vi "PIL_GUI_Fake.vi"() -> ()   [LabVIEW 2015]
doc: "Utilisez ce modèle pour construire un modèle de conception Machine à états standard. Chaque état exécute du code et détermine l'état suivant à exécuter."
uses:
  QMH_MessageCluster.ctl
panel:
  in  "Commande onglets":enum32{"Experiment", "Hardware"}(tab)
  out "error out":errorcluster
  in  "error in (no error)":errorcluster
  out "Consumer State":string
  in  "Exit":bool caption="Stop"
  in  "Save":bool caption="Stop"
  in  "Load":bool caption="Stop"
  in  "Stop":bool
  in  "Settings":bool caption="Record"
  in  "Play":bool
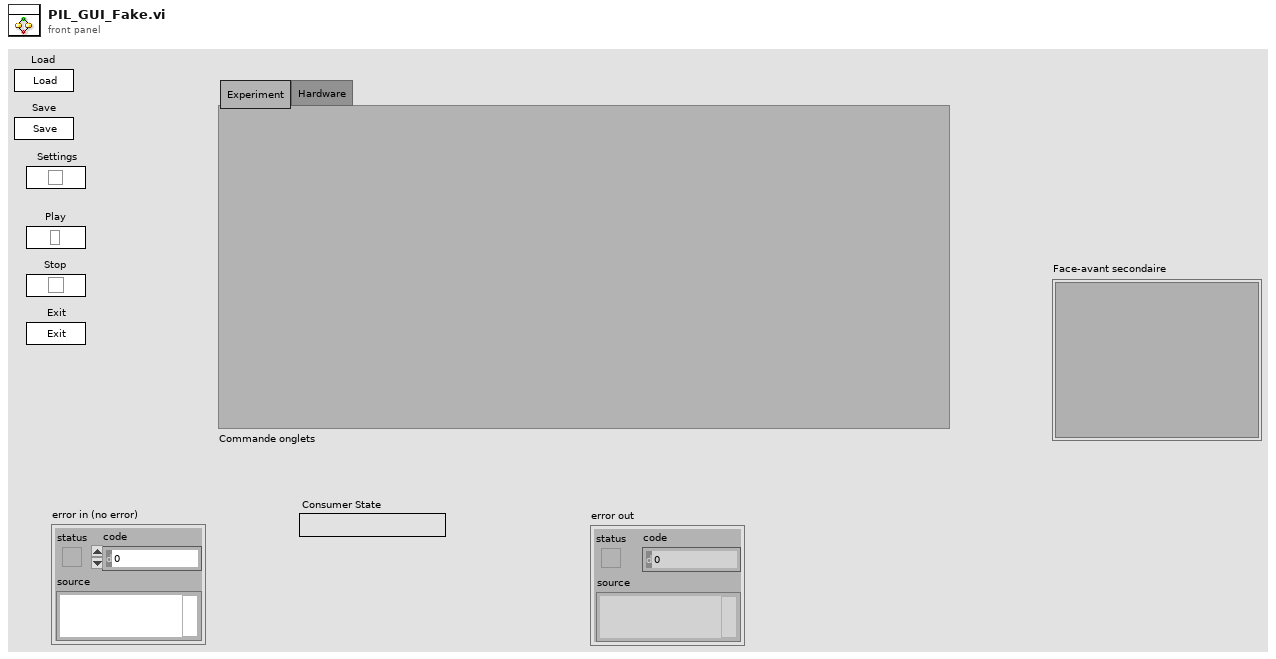
[diagram p1: front panel]
types:
  T1 = enum16{"Initialize", "Settings", "Load", "Save", "Play", "Stop", "Exit"}
  T2 = typedef "QMH_MessageCluster.ctl" = cluster{"Command":enum16{"Initialize", "Settings", "Load", "Save", "Play", "Stop", "Exit"}, "Data":variant}
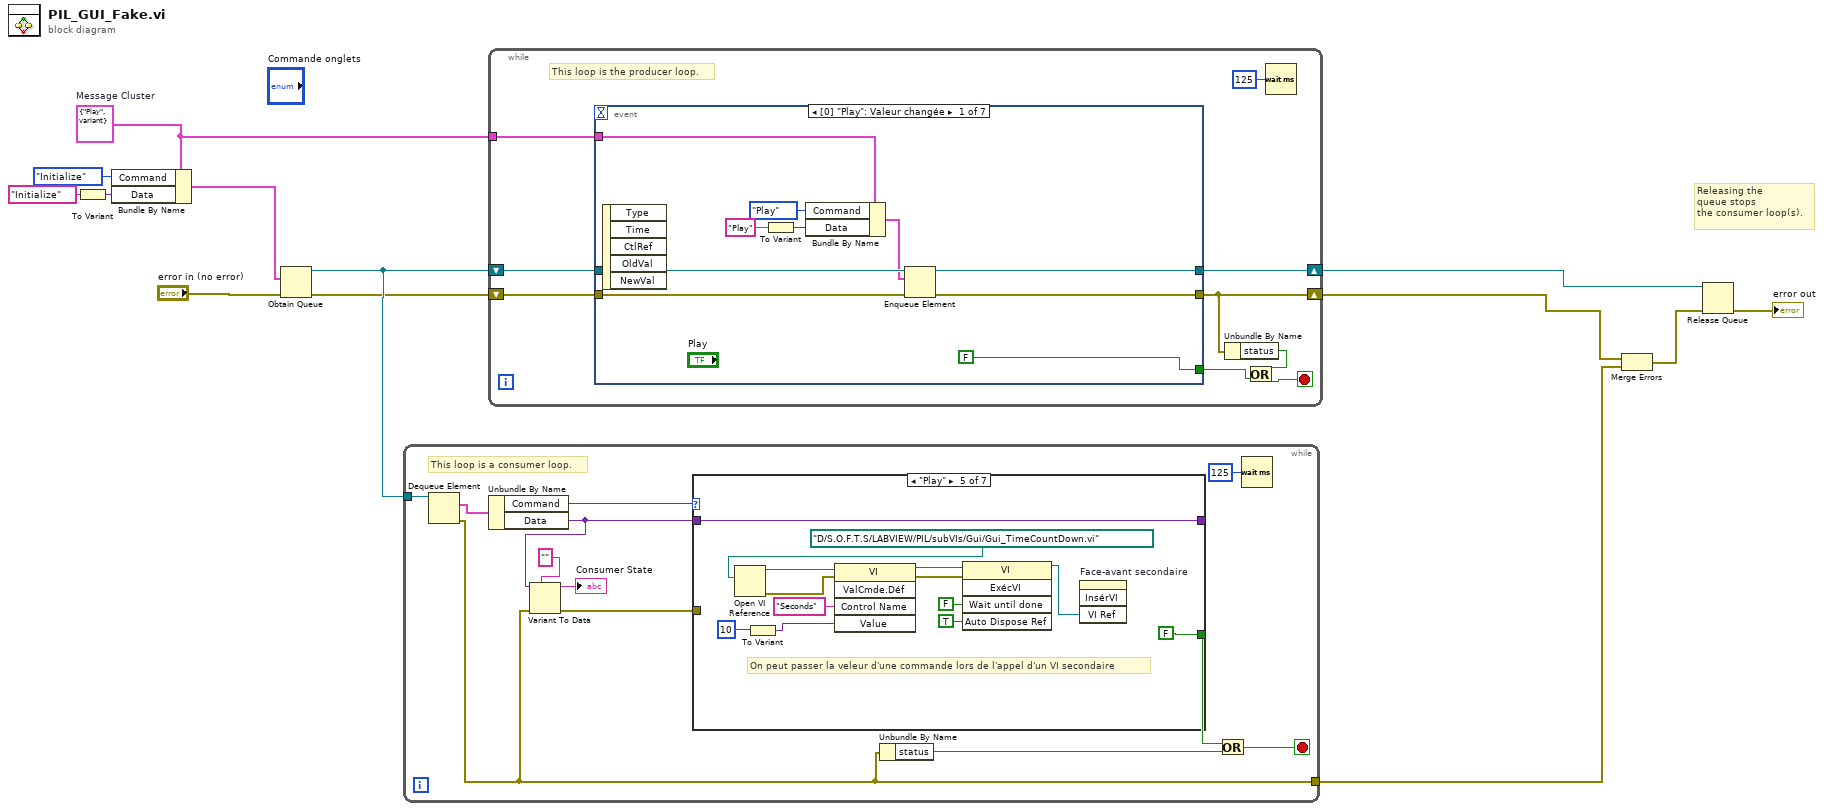
[diagram p0: block diagram]
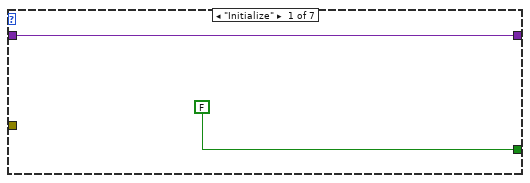
[diagram p2: hidden frame]
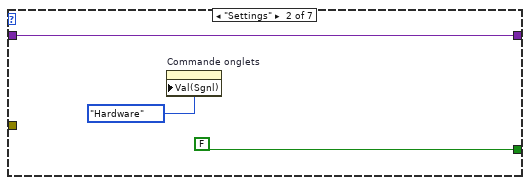
[diagram p3: hidden frame]
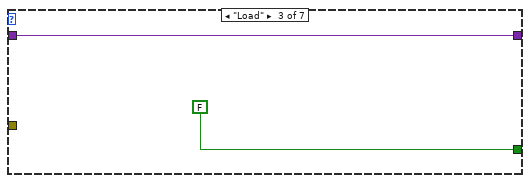
[diagram p4: hidden frame]
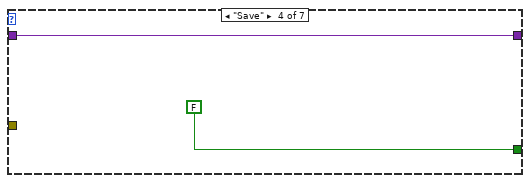
[diagram p5: hidden frame]
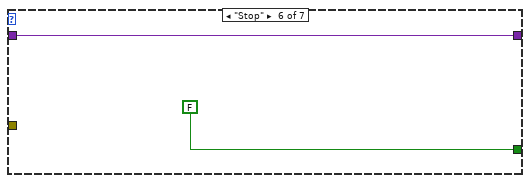
[diagram p6: hidden frame]
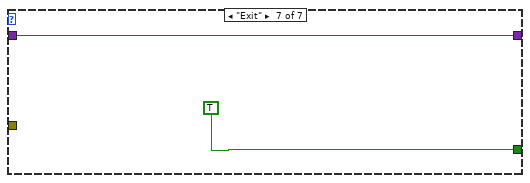
[diagram p7: hidden frame]
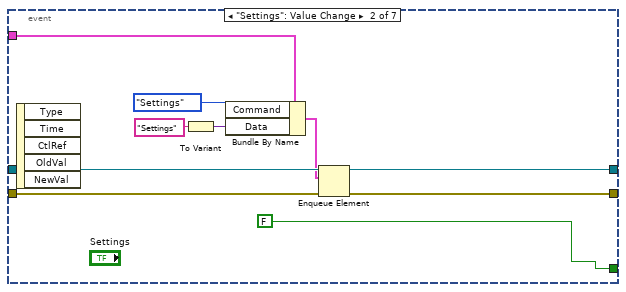
[diagram p8: hidden frame]
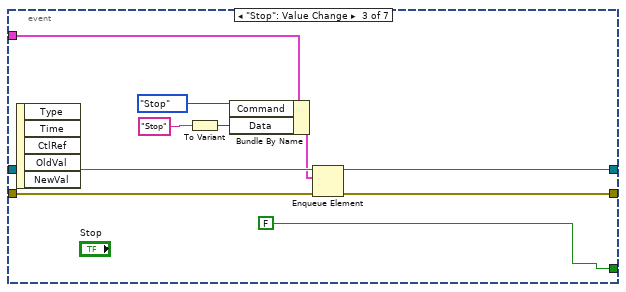
[diagram p9: hidden frame]
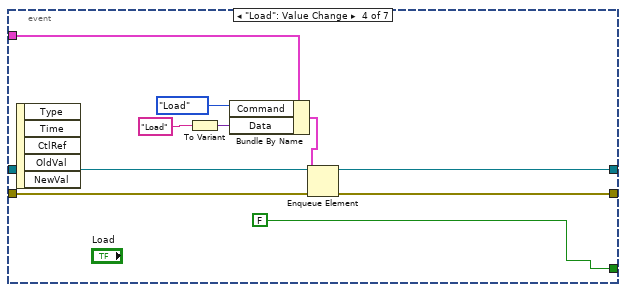
[diagram p10: hidden frame]
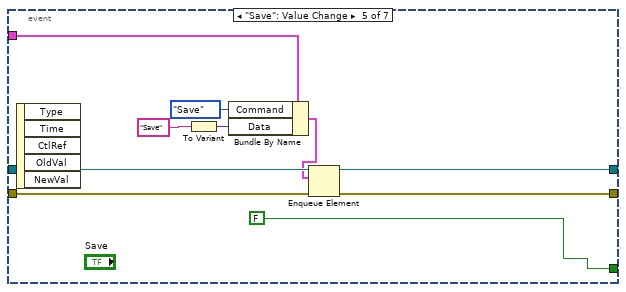
[diagram p11: hidden frame]
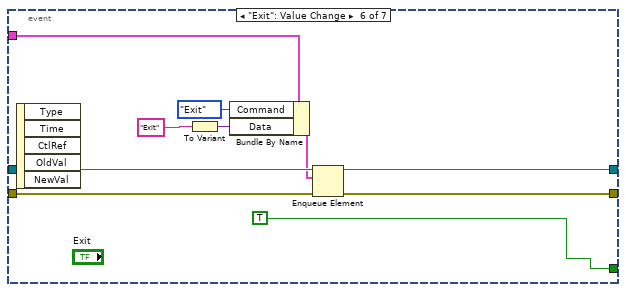
[diagram p12: hidden frame]
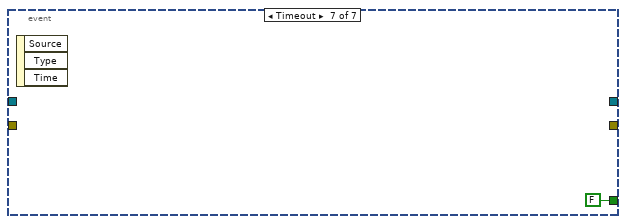
[diagram p13: hidden frame]
diagram:
  w2 = T2 {"Command"=enum."Play", "Data"=variant}  # Message Cluster
  # "Releasing the\nqueue stops\nthe consumer loop(s)."
  n1 = To Variant(anything="Initialize") -> (Variant=w4:variant)
  n2 = Bundle By Name(cluster=w2, "Command"=T1."Initialize", "Data"=w4) -> (w3:T2)
  n3 = Obtain Queue(element data type=w3, error in (no error)="error in (no error)") -> (queue out=w13:refnum<queue>, error out=w12:errorcluster)  [unwired: 2 in, 2 out]
  n4 = while {
    tunnel: w13 -> [w24]
    tunnel: [w20] -> w6
    stop <- w16 stop-if-true
    # "This loop is a consumer loop."
    n5 = Dequeue Element(queue=w24) -> (element=w19:T2, error out=w20:errorcluster)  [unwired: 1 in, 3 out]
    n6 = Unbundle By Name(w19) -> ("Command"=w14:T1, "Data"=w15:variant)
    n7 = Variant To Data(type="", Variant=w15) -> (data=→"Consumer State":string)  [unwired: 1 in, 1 out]
    n8 = case shown="\"Play\"" w14 {
      tunnel: [w25 w28 w30 w32 w45 w47 w49] -> _
      tunnel: [FALSE ("x") FALSE ("x") FALSE ("x") FALSE ("x") FALSE ("x") FALSE ("x") TRUE ("x")] -> w22
      tunnel: w15 -> [w25 w28 w30 w32 w45 w47 w49]
      tunnel: w20 -> [_ _ _ _ _ _ _]
      frame "Initialize" {
      }
      frame "Settings" {
        n9 = property on="Commande onglets" class="Onglet (strict)"("Val(Sgnl)"=enum32{"Experiment", "Hardware"}."Hardware" ("Commande onglets")) -> ()  [unwired: 2 in, 2 out]
      }
      frame "Load" {
      }
      frame "Save" {
      }
      frame "Play" {
        # "On peut passer la veleur d'une commande lors de l'appel d'un VI secondaire"
        n10 = Open VI Reference(vi path=path "D:/S.O.F.T.S/LABVIEW/PIL/subVIs/Gui/Gui_TimeCountDown.vi" ("chemin du VI")) -> (vi reference=w41:refnum<vi>, error out=w39:errorcluster)  [unwired: 5 in]
        n11 = To Variant(anything=10) -> (Variant=w35:variant)
        n12 = invoke class="VI" method="ValCmde.Déf"(reference=w41, error in=w39, "Control Name"="Seconds" ("Nom de la commande"), "Value"=w35) -> (reference out=w40:refnum<vi>, error out=w38:errorcluster)  [unwired: 1 in, 3 out]
        n13 = invoke class="VI" method="ExécVI"(reference=w40, error in=w38, "Wait until done"=FALSE ("Attendre la fin"), "Auto Dispose Ref"=TRUE ("Supprimer la référence automatiquement")) -> (reference out=w42:refnum<vi>)  [unwired: 1 in, 4 out]
        n14 = invoke on="Face-avant secondaire" class="FAsec" method="InsérVI"("VI Ref"=w42) -> ()  [unwired: 3 in, 4 out]
      }
      frame "Stop" {
      }
      frame "Exit" {
      }
    }
    n15 = Unbundle By Name(w20) -> ("status"=w23:bool)
    n16 = Or(x=w22, y=w23) -> (x .or. y?=w16:bool)
    n17 = Wait (ms)(milliseconds to wait=u32 125) -> ()  [unwired: 1 out]
  }
  n18 = while {
    shift-right: [w55] -> w7
    shift-left: w12 -> [w56]
    shift-right: [w54] -> w11
    shift-left: w13 -> [w57]
    tunnel: w2 -> [w52]
    stop <- w59 stop-if-true
    # "This loop is the producer loop."
    n19 = event shown="[0] \"Play\": Valeur changée" {
      selector: _ -> [_ _ _ _ _ _ _]
      dyn-events: _ -> [_ _ _ _ _ _ _]
      timeout: _ -> [_ _ _ _ _ _ _]
      tunnel: w57 -> [w69 w79 w89 w99 w109 w119 _]
      tunnel: w56 -> [w68 w78 w88 w98 w108 w118 _]
      tunnel: [w67 w77 w87 w97 w107 w117 _] -> w55
      tunnel: [w66 w76 w86 w96 w106 w116 _] -> w54
      tunnel: [FALSE ("Stop") FALSE ("Stop") FALSE ("Stop") FALSE ("Stop") FALSE ("Stop") TRUE ("Stop") FALSE ("Stop")] -> w53
      tunnel: w52 -> [w62 w72 w82 w92 w102 w112 _]
      event "Play": Value Change {
        n20 = event-data() -> ()  [unwired: 6 out]
        n21 = To Variant(anything="Play") -> (Variant=w63:variant)
        n22 = Bundle By Name(cluster=w62, "Command"=T1."Play", "Data"=w63) -> (w61:T2)
        n23 = Enqueue Element(queue=w69, element=w61, error in (no error)=w68) -> (queue out=w66:refnum<queue>, error out=w67:errorcluster)  [unwired: 2 out]
      }
      event "Settings": Value Change {
        n24 = event-data() -> ()  [unwired: 6 out]
        n25 = To Variant(anything="Settings") -> (Variant=w74:variant)
        n26 = Bundle By Name(cluster=w72, "Command"=T1."Settings", "Data"=w74) -> (w71:T2)
        n27 = Enqueue Element(queue=w79, element=w71, error in (no error)=w78) -> (queue out=w76:refnum<queue>, error out=w77:errorcluster)  [unwired: 2 out]
      }
      event "Stop": Value Change {
        n28 = event-data() -> ()  [unwired: 6 out]
        n29 = To Variant(anything="Stop") -> (Variant=w84:variant)
        n30 = Bundle By Name(cluster=w82, "Command"=T1."Stop", "Data"=w84) -> (w81:T2)
        n31 = Enqueue Element(queue=w89, element=w81, error in (no error)=w88) -> (queue out=w86:refnum<queue>, error out=w87:errorcluster)  [unwired: 2 out]
      }
      event "Load": Value Change {
        n32 = event-data() -> ()  [unwired: 6 out]
        n33 = To Variant(anything="Load") -> (Variant=w94:variant)
        n34 = Bundle By Name(cluster=w92, "Command"=T1."Load", "Data"=w94) -> (w91:T2)
        n35 = Enqueue Element(queue=w99, element=w91, error in (no error)=w98) -> (queue out=w96:refnum<queue>, error out=w97:errorcluster)  [unwired: 2 out]
      }
      event "Save": Value Change {
        n36 = event-data() -> ()  [unwired: 6 out]
        n37 = To Variant(anything="Save") -> (Variant=w104:variant)
        n38 = Bundle By Name(cluster=w102, "Command"=T1."Save", "Data"=w104) -> (w101:T2)
        n39 = Enqueue Element(queue=w109, element=w101, error in (no error)=w108) -> (queue out=w106:refnum<queue>, error out=w107:errorcluster)  [unwired: 2 out]
      }
      event "Exit": Value Change {
        n40 = event-data() -> ()  [unwired: 6 out]
        n41 = To Variant(anything="Exit") -> (Variant=w114:variant)
        n42 = Bundle By Name(cluster=w112, "Command"=T1."Exit", "Data"=w114) -> (w111:T2)
        n43 = Enqueue Element(queue=w119, element=w111, error in (no error)=w118) -> (queue out=w116:refnum<queue>, error out=w117:errorcluster)  [unwired: 2 out]
      }
      event Timeout {
        n44 = event-data() -> ()  [unwired: 4 out]
      }
    }
    n45 = Unbundle By Name(w55) -> ("status"=w58:bool)
    n46 = Or(x=w58, y=w53) -> (x .or. y?=w59:bool)
    n47 = Wait (ms)(milliseconds to wait=u32 125) -> ()  [unwired: 1 out]
  }
  n48 = Merge Errors(w7, w6) -> (w8:errorcluster)
  n49 = Release Queue(queue=w11, error in (no error)=w8) -> (error out=→"error out":errorcluster)  [unwired: 3 out]
